vi "102_Lipgap_Full_Algo_old.vi"(0 "Image":T3(plugin-control), 1 "Calibrated Image":T3, 2 "Reference ROI":T1 {"Contours"."Type" items=["No Selection", "Point", "Line", "Rectangle", "Oval", "Polygon", "Freehand Region", "Annulus", "Unused2", "Unused3", "Broken Line", "Freehand Line", "Rotated Rectangle"]}, 3 "Line Options ROI Ref":T7={"Number of Lines"=1, "Type"=enum."First Edge Rake", "Min. Score"=10.0, "Max. Score"=1000.0, "Orientation"=0.0, "Angle Range"=45.0, "Angle Tolerance"=1.0, "Step Size"=3, "Min. SNR (db)"=0.0, "Min. Points (%)"=25.0, "Hough Iterations"=5} {"Min. Points (%)" min=0.0 max=100.0; "Min. SNR (db)" min=0.0; "Max. Score" min=0.0 max=1024.0; "Min. Score" min=0.0 max=1024.0 step=1.0}, 4 "Edge Options ROI Ref":T4={"Edge Polarity"=0, "Kernel Size"=3, "Width"=3, "Minimum Edge Strength"=50.0, "Interpolation Type"=enum."Zero Order", "Data Processing Method"=enum."Average"} {"Edge Polarity" items=["All Edges", "Rising Edges", "Falling Edges"]; "Minimum Edge Strength" format="%.2f"; "Width" step=2; "Kernel Size" step=2}, 5 "Search Direction ROI Ref":u32=3, 6 "Measurement ROI 1":T1 {"Contours"."Type" items=["No Selection", "Point", "Line", "Rectangle", "Oval", "Polygon", "Freehand Region", "Annulus", "Unused2", "Unused3", "Broken Line", "Freehand Line", "Rotated Rectangle"]}, 7 "error in (no error)":errorcluster, 8 "Blob Center":cluster{"Center X":dbl, "Center Y":dbl}, 9 "Search Direction ROI 1":u16(ring)=2 items=["Left To Right", "Right To Left", "Top To Bottom", "Bottom To Top"], 10 "Edge Options ROI 1":T4={"Edge Polarity"=0, "Kernel Size"=3, "Width"=3, "Minimum Edge Strength"=50.0, "Interpolation Type"=enum."Zero Order", "Data Processing Method"=enum."Average"} {"Edge Polarity" items=["All Edges", "Rising Edges", "Falling Edges"]; "Minimum Edge Strength" format="%.2f"; "Width" step=2; "Kernel Size" step=2}, 11 "Measurement ROI 2":T1 {"Contours"."Type" items=["No Selection", "Point", "Line", "Rectangle", "Oval", "Polygon", "Freehand Region", "Annulus", "Unused2", "Unused3", "Broken Line", "Freehand Line", "Rotated Rectangle"]}, 13 "Edge Options ROI 2":T4={"Edge Polarity"=0, "Kernel Size"=3, "Width"=3, "Minimum Edge Strength"=10.0, "Interpolation Type"=enum."Bilinear Fixed", "Data Processing Method"=enum."Average"} {"Edge Polarity" items=["All Edges", "Rising Edges", "Falling Edges"]; "Minimum Edge Strength" format="%.2f"; "Width" step=2; "Kernel Size" step=2}, 14 "Process ROI 2":T6(ring)=enum."Get All Edges", 15 "Step Size ROI 2":u32=5) -> (20 "Real World Lip Gap 102":sgl, 21 "102 Lip Gap cluster out":T2 {"102 Lip Gap ROI out"."Contours"."Type" items=["No Selection", "Point", "Line", "Rectangle", "Oval", "Polygon", "Freehand Region", "Annulus", "Unused2", "Unused3", "Broken Line", "Freehand Line", "Rotated Rectangle"]}, 27 "error IO":errorcluster)   [LabVIEW 2015]
uses:
  <vilib>/vision/Measure.llb/Straight Edge Options.ctl
  <vilib>/vision/Measure.llb/Straight Edge Process.ctl
  <vilib>/vision/Measure.llb/Edge Options.ctl
  <vilib>/vision/Measure.llb/Edge Polarity.ctl
  <vilib>/vision/Image Controls.llb/IMAQ Image.ctl
  SubVI/Clamp.llb/Find Min Max Position.vi
  <vilib>/vision/NI_Vision_Development_Module.lvlib
  FrameworkOverrides/Algorithm.lvclass
panel:
  out "Array":i32[](array[numeric])
  out "min value":sgl
  out "max value":sgl
  out "x/y":sgl
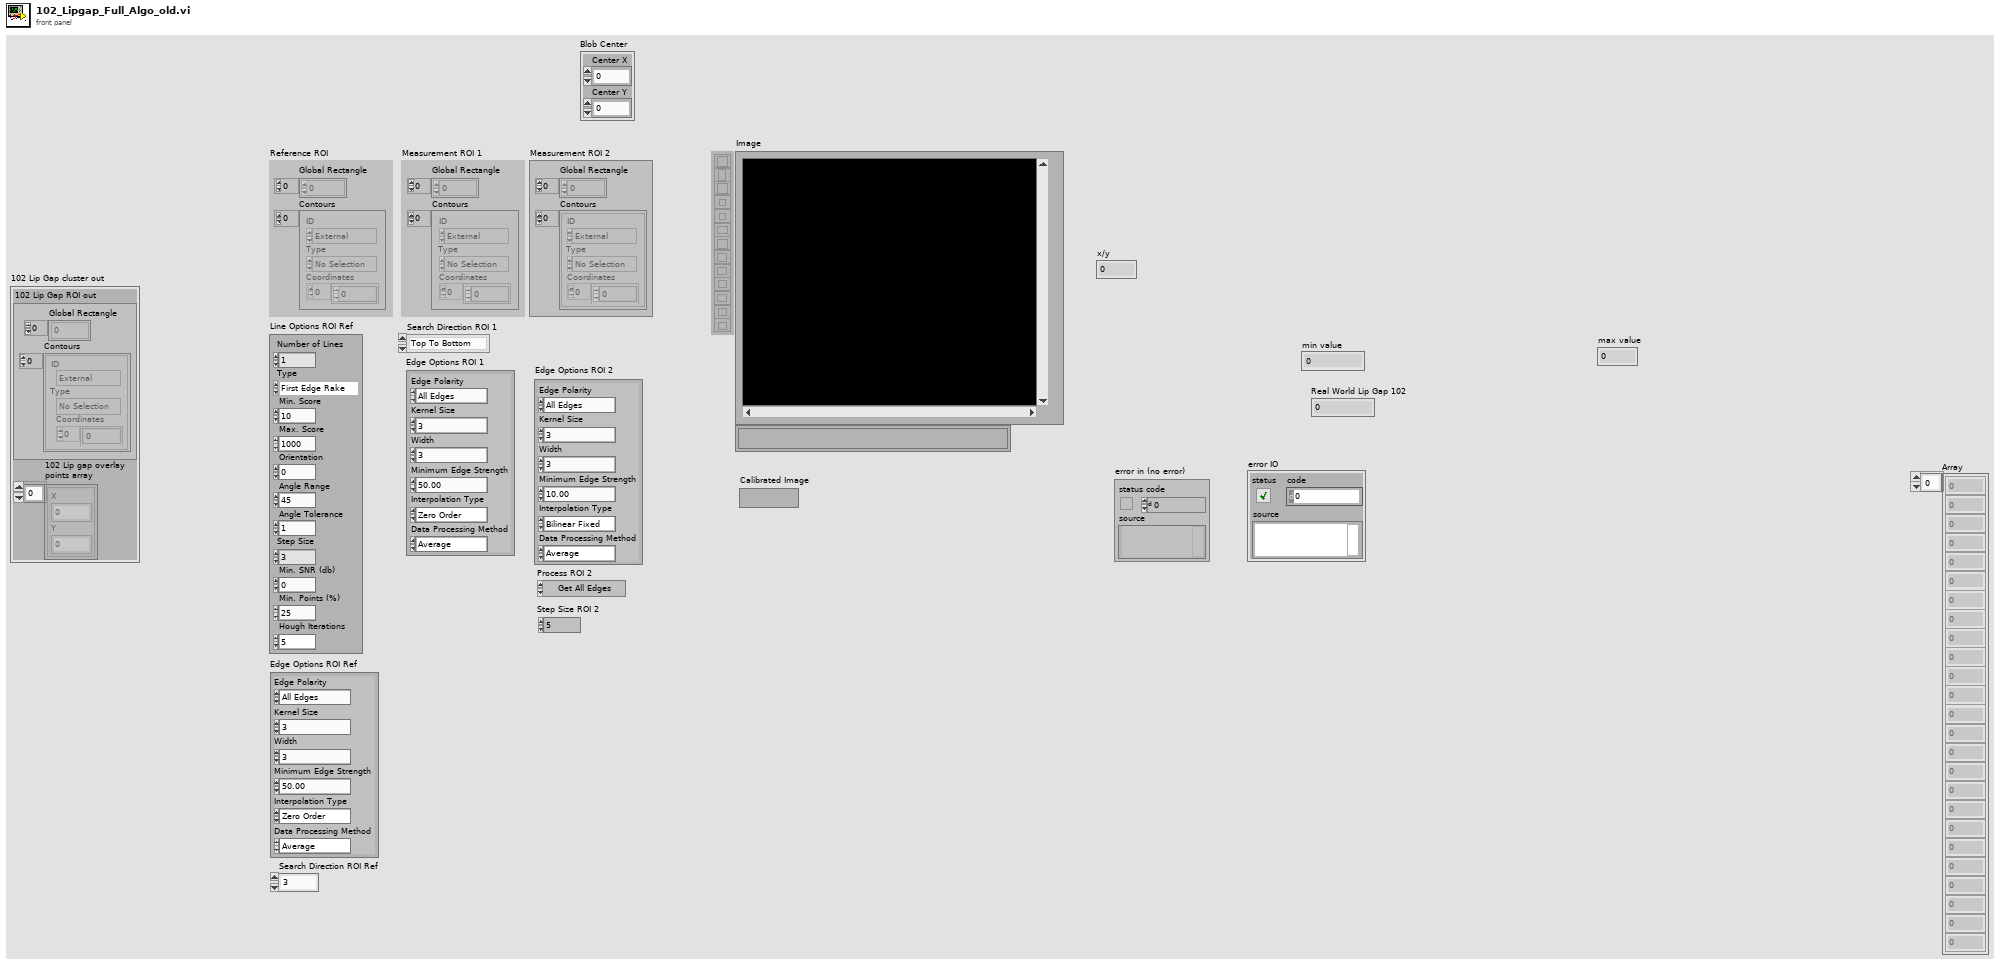
[diagram p1: front panel]
types:
  T1 = typedef "ROI Descriptor" = cluster{"Global Rectangle":i32[], "Contours":cluster{"ID":enum32{"External", "Internal"}, "Type":u32, "Coordinates":i32[]}[]}
  T2 = cluster{"102 Lip Gap ROI out":T1, "102 Lip gap overlay\npoints array":cluster{"X":sgl, "Y":sgl}[]}
  T3 = typedef "IMAQ Image.ctl" = refnum<image>
  T4 = typedef "Edge Options.ctl" = cluster{"Edge Polarity":T5, "Kernel Size":u32, "Width":u32, "Minimum Edge Strength":sgl, "Interpolation Type":enum32{"Zero Order", "Bilinear", "Quadratic", "Cubic", "Bilinear Fixed"}, "Data Processing Method":enum32{"Average", "Median"}}
  T5 = typedef "Edge Polarity.ctl" = u32
  T6 = enum16{"Get First Edge", "Get First + Last Edge", "Get All Edges", "Get Best Edge"}
  T7 = typedef "Straight Edge Options.ctl" = cluster{"Number of Lines":i32, "Type":T8, "Min. Score":dbl, "Max. Score":dbl, "Orientation":dbl, "Angle Range":dbl, "Angle Tolerance":dbl, "Step Size":u32, "Min. SNR (db)":dbl, "Min. Points (%)":dbl, "Hough Iterations":i32}
  T8 = typedef "Straight Edge Process.ctl" = enum32{"First Edge Rake", "Best Edge Rake", "Hough Edge Rake", "First Edge Projection", "Best Edge Projection"}
  T9 = typedef "IMAQ Rectangle" = cluster{"Left":i32, "Top":i32, "Right":i32, "Bottom":i32, "Rotation":dbl}
  T10 = cluster{"Left":dbl, "Top":dbl, "Right":dbl, "Bottom":dbl, "Angle":dbl}
  T11 = cluster{"Search Direction":u32, "Edge Options":T4, "Show Search Area":bool, "Show Search Lines":bool, "Show Edges Found":bool, "Show Result":bool, "Search Area Color":u32, "Search Lines Color":u32, "Edge Locations Color":u32, "Result Color":u32, "Overlay Group Name":string}
  T12 = cluster{"Point1 (Pixels)":cluster{"X":sgl, "Y":sgl}, "Point2 (Pixels)":cluster{"X":sgl, "Y":sgl}, "Point1 (Real-World)":cluster{"X":sgl, "Y":sgl}, "Point2 (Real-World)":cluster{"X":sgl, "Y":sgl}, "Angle (Pixel)":dbl, "Angle (Real-World)":dbl, "Score":dbl, "Straightness":dbl, "Average SNR (db)":dbl, "Calibration Valid":bool}[]
  T13 = cluster{"Point1 (Pixels)":cluster{"X":sgl, "Y":sgl}, "Point2 (Pixels)":cluster{"X":sgl, "Y":sgl}, "Point1 (Real-World)":cluster{"X":sgl, "Y":sgl}, "Point2 (Real-World)":cluster{"X":sgl, "Y":sgl}, "Angle (Pixel)":dbl, "Angle (Real-World)":dbl, "Score":dbl, "Straightness":dbl, "Average SNR (db)":dbl, "Calibration Valid":bool}
  T14 = typedef "IMAQ Line" = cluster{"Start X":i32, "Start Y":i32, "End X":i32, "End Y":i32}
  T15 = typedef "Search Line.ctl" = cluster{"Start Point":cluster{"X":sgl, "Y":sgl}, "End Point":cluster{"X":sgl, "Y":sgl}, "Edge Info":T16[], "Edge Map":dbl[], "Calibration Valid":bool}
  T16 = typedef "Edge New.ctl" = cluster{"Location (Pixel)":cluster{"X":sgl, "Y":sgl}, "Location (Real-World)":cluster{"X":sgl, "Y":sgl}, "Distance (Pixel)":dbl, "Distance (Real-World)":dbl, "Strength":dbl, "Noise":dbl, "Rising?":bool}
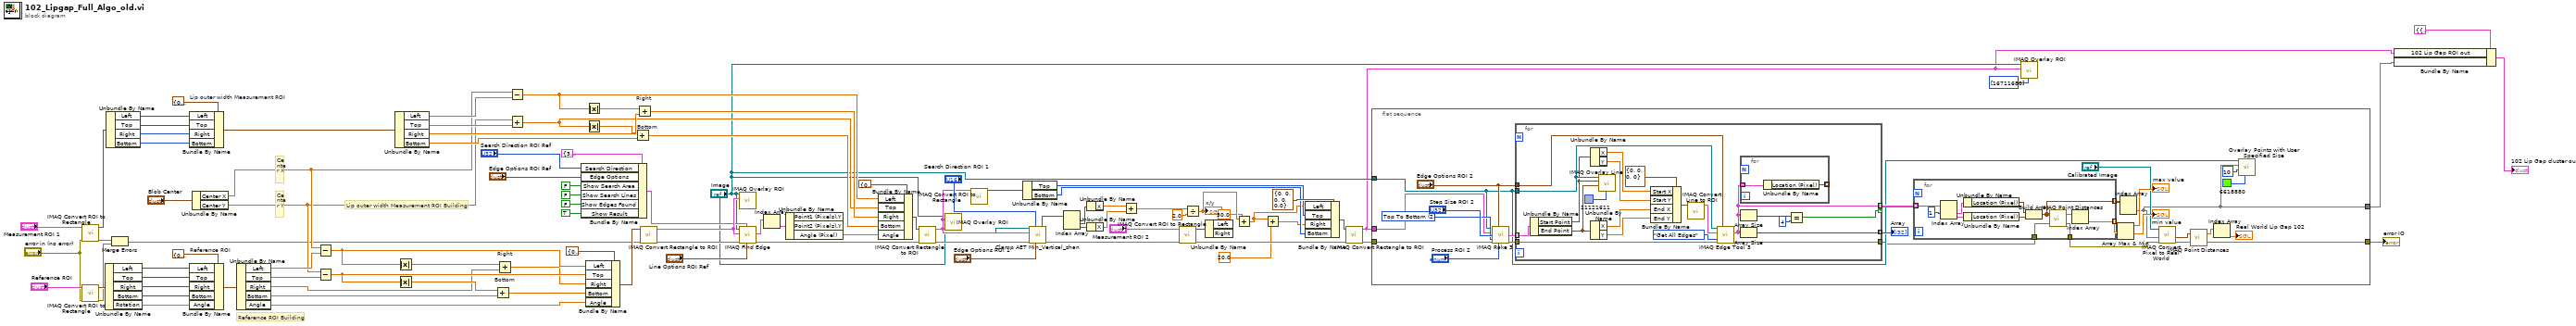
[diagram p0: block diagram]
diagram:
  # "Lip outer width Measurement ROI Building"
  # "Reference ROI Building"
  # "Center Y"
  # "Center X"
  n1 = call "IMAQ Convert ROI to Rectangle"("error in (no error)"="error in (no error)", "ROI Descriptor"="Measurement ROI 1") -> ("error out"=w45:errorcluster, "Rectangle"=w56:T9)  [unwired: 7 in]
  n2 = call "IMAQ Convert ROI to Rectangle"("error in (no error)"="error in (no error)", "ROI Descriptor"="Reference ROI") -> ("error out"=w44:errorcluster, "Rectangle"=w51:T9)  [unwired: 7 in]
  n3 = Unbundle By Name(w51) -> ("Left"=w50:i32, "Top"=w49:i32, "Right"=w48:i32, "Bottom"=w47:i32, "Rotation"=w46:dbl)
  n4 = Unbundle By Name(w56) -> ("Left"=w55:i32, "Top"=w54:i32, "Right"=w53:i32, "Bottom"=w52:i32)
  n5 = Merge Errors(w45, w44) -> (w43:errorcluster)
  n6 = Bundle By Name "Lip outer width Measurement ROI"(cluster=T10 {"Left"=0.0, "Top"=0.0, "Right"=0.0, "Bottom"=0.0, "Angle"=0.0} ("input cluster"), "Left"=w55, "Top"=w54, "Right"=w53, "Bottom"=w52) -> (w64:T10)
  n7 = Bundle By Name "Reference ROI"(cluster=T10 {"Left"=0.0, "Top"=0.0, "Right"=0.0, "Bottom"=0.0, "Angle"=0.0} ("input cluster"), "Left"=w50, "Top"=w49, "Right"=w48, "Bottom"=w47, "Angle"=w46) -> (w63:T10)
  n8 = Unbundle By Name("Blob Center") -> ("Center X"=w58:dbl, "Center Y"=w57:dbl)
  n9 = Unbundle By Name(w63) -> ("Left"=w90:dbl, "Top"=w89:dbl, "Right"=w88:dbl, "Bottom"=w87:dbl, "Angle"=w86:dbl)
  n10 = Subtract(x=w58, y=w90) -> (x-y=w94:dbl)
  n11 = Subtract(x=w57, y=w89) -> (x-y=w93:dbl)
  n12 = Unbundle By Name(w64) -> ("Left"=w73:dbl, "Top"=w72:dbl, "Right"=w71:dbl, "Bottom"=w70:dbl)
  n13 = Absolute Value(x=w94) -> (abs(x)=w97:dbl)
  n14 = Absolute Value(x=w93) -> (abs(x)=w96:dbl)
  n15 = Add "Bottom"(x=w96, y=w87) -> (x+y=w91:dbl)
  n16 = Add "Right"(x=w97, y=w88) -> (x+y=w92:dbl)
  n17 = Subtract(x=w58, y=w73) -> (x-y=w76:dbl)
  n18 = Add(x=w57, y=w72) -> (x+y=w68:dbl)
  n19 = Bundle By Name(cluster=T11 {"Search Direction"=3, "Edge Options"={"Edge Polarity"=0, "Kernel Size"=3, "Width"=3, "Minimum Edge Strength"=50.0, "Interpolation Type"=enum."Zero Order", "Data Processing Method"=enum."Average"}, "Show Search Area"=FALSE, "Show Search Lines"=FALSE, "Show Edges Found"=FALSE, "Show Result"=TRUE, "Search Area Color"=65280, "Search Lines Color"=255, "Edge Locations Color"=16776960, "Result Color"=16711680, "Overlay Group Name"=""} ("Options"), "Search Direction"="Search Direction ROI Ref", "Edge Options"="Edge Options ROI Ref", "Show Search Area"=FALSE, "Show Search Lines"=FALSE, "Show Edges Found"=FALSE, "Show Result"=TRUE) -> (w38:T11)
  n20 = Absolute Value(x=w76) -> (abs(x)=w78:dbl)
  n21 = Absolute Value(x=w68) -> (abs(x)=w69:dbl)
  n22 = Bundle By Name(cluster=T10 {"Left"=0.0, "Top"=0.0, "Right"=0.0, "Bottom"=0.0, "Angle"=0.0} ("input cluster"), "Left"=w94, "Top"=w93, "Right"=w92, "Bottom"=w91, "Angle"=w86) -> (w81:T10)
  n23 = Add "Bottom"(x=w69, y=w70) -> (x+y=w74:dbl)
  n24 = Add "Right"(x=w78, y=w71) -> (x+y=w75:dbl)
  n25 = call "IMAQ Convert Rectangle to ROI"("error in (no error)"=w43, "Rectangle"=w81) -> ("error out"=w85:errorcluster, "ROI Descriptor"=w79:T1)  [unwired: 7 in]
  n26 = call "IMAQ Overlay ROI"("ROI Descriptor"=w79, "Image"="Image") -> ()  [unwired: 8 in, 2 out]
  n27 = call "IMAQ Find Edge"("Line Fit Options"="Line Options ROI Ref", "Options"=w38, "error in (no error)"=w85, "ROI Descriptor"=w79, "Image"="Image") -> ("error out"=w42:errorcluster, "Straight Edges"=w83:T12)  [unwired: 3 in, 2 out]
  n28 = Index Array(array=w83) -> (element=w82:T13)  [unwired: 1 in]
  n29 = Unbundle By Name(w82) -> ("Angle (Pixel)"=w66:dbl)  [unwired: 2 out]
  n30 = Bundle By Name(cluster=T10 {"Left"=0.0, "Top"=0.0, "Right"=0.0, "Bottom"=0.0, "Angle"=0.0} ("input cluster"), "Left"=w76, "Top"=w68, "Right"=w75, "Bottom"=w74, "Angle"=w66) -> (w67:T10)
  n31 = call "IMAQ Convert Rectangle to ROI"("error in (no error)"=w42, "Rectangle"=w67) -> ("error out"=w62:errorcluster, "ROI Descriptor"=w23:T1)  [unwired: 7 in]
  n32 = call "IMAQ Overlay ROI"("ROI Descriptor"=w23, "Image"="Image") -> ()  [unwired: 8 in, 2 out]
  n33 = call "IMAQ Convert ROI to Rectangle"("ROI Descriptor"=w23) -> ("Rectangle"=w22:T9)  [unwired: 8 in, 1 out]
  n34 = Unbundle By Name(w22) -> ("Top"=w20:i32, "Bottom"=w19:i32)
  n35 = call "Clamp AET Min_Vertical_shan.vi"("Image"="Image", "Scanning axis"="Search Direction ROI 1", "ROI Descriptor"=w23, "error in (no error)"=w62, "Edge Options"="Edge Options ROI 1") -> ("Edge Coordinates"=w31:cluster{"X":sgl, "Y":sgl}[], "error out"=w10:errorcluster)  [unwired: 3 in, 6 out]
  n36 = Index Array(array=w31) -> (element #1=w30:cluster{"X":sgl, "Y":sgl}, element #2=w29:cluster{"X":sgl, "Y":sgl})  [unwired: 2 in]
  n37 = Unbundle By Name(w30) -> ("X"=w28:sgl)
  n38 = Unbundle By Name(w29) -> ("X"=w27:sgl)
  n39 = Add(x=w28, y=w27) -> (x+y=w26:sgl)
  n40 = call "IMAQ Convert ROI to Rectangle"("error in (no error)"=w10, "ROI Descriptor"="Measurement ROI 2") -> ("error out"=w9:errorcluster, "Rectangle"=w12:T9)  [unwired: 7 in]
  n41 = Divide(x=w26, y=sgl 2.0) -> (x/y=w24:sgl)
  "x/y" <- w24
  n42 = Unbundle By Name(w12) -> ()  [unwired: 2 out]
  n43 = Add(x=w24, y=sgl 30.0) -> (x+y=w18:sgl)
  n44 = Add(x=w18, y=sgl 20.0) -> (x+y=w17:sgl)
  n45 = Bundle By Name(cluster=T9 {"Left"=0, "Top"=0, "Right"=0, "Bottom"=0, "Rotation"=0.0} ("Rectangle"), "Left"=w18, "Top"=w20, "Right"=w17, "Bottom"=w19) -> (w16:T9)
  n46 = call "IMAQ Convert Rectangle to ROI"("error in (no error)"=w9, "Rectangle"=w16) -> ("error out"=w13:errorcluster, "ROI Descriptor"=w2:T1)  [unwired: 7 in]
  n47 = flat-sequence {
    tunnel: "Image" -> [w101]
    tunnel: w2 -> [w107]
    tunnel: w13 -> [w106]
    tunnel: [w104] -> w7
    tunnel: [w98] -> w1
    frame #0 {
      w122 = u16 2 items=["Left To Right", "Right To Left", "Top To Bottom", "Bottom To Top"] ("Scan Direction ROI 2")
      n48 = call "IMAQ Rake 3"("Image"=w101, "Edge Options"="Edge Options ROI 2", "ROI Descriptor"=w107, "Step Size"="Step Size ROI 2", "Scan Direction"=w122, "error in (no error)"=w106, "Process"="Process ROI 2") -> ("Search Lines"=w120:T15[], "error out"=w118:errorcluster)  [unwired: 5 in, 2 out]
      n49 = for {
        tunnel: w120 -> [w155] mode=indexing
        tunnel: w101 -> [w144]
        tunnel: "Edge Options ROI 2" -> [w145]
        tunnel: w118 -> [w143]
        tunnel: [w142] -> w100
        tunnel: [w139] -> w117 mode=indexing
        tunnel: [w138] -> w116 mode=indexing if=w135
        n50 = Unbundle By Name(w155) -> ("Start Point"=w141:cluster{"X":sgl, "Y":sgl}, "End Point"=w140:cluster{"X":sgl, "Y":sgl})
        n51 = Unbundle By Name(w141) -> ("X"=w152:sgl, "Y"=w151:sgl)
        n52 = Unbundle By Name(w140) -> ("X"=w150:sgl, "Y"=w149:sgl)
        n53 = call "IMAQ Overlay Line"("Color"=u32 11121611, "End Point"=w140, "Start Point"=w141, "Image"=w144) -> ()  [unwired: 6 in, 2 out]
        n54 = Bundle By Name(cluster=T14 {"Start X"=0, "Start Y"=0, "End X"=0, "End Y"=0} ("Line"), "Start X"=w152, "Start Y"=w151, "End X"=w150, "End Y"=w149) -> (w148:T14)
        n55 = call "IMAQ Convert Line to ROI"("Line"=w148) -> ("ROI Descriptor"=w147:T1)  [unwired: 8 in, 1 out]
        n56 = call "IMAQ Edge Tool 3"("Image"=w144, "Edge Options"=w145, "ROI Descriptor"=w147, "Process"=T6."Get All Edges", "error in (no error)"=w143) -> ("Edge Information"=w138:T16[], "error out"=w142:errorcluster)  [unwired: 6 in, 3 out]
        n57 = for {
          tunnel: w138 -> [w157] mode=indexing
          tunnel: [w156] -> _ mode=indexing
          n58 = Unbundle By Name(w157) -> ("Location (Pixel)"=w156:cluster{"X":sgl, "Y":sgl})
        }
        n59 = Array Size(array=w138) -> (size(s)=w137:i32)
        n60 = Array Size(array=w138) -> (size(s)=w139:i32)
        n61 = Equal?(x=w137, y=4) -> (x = y?=w135:bool)
      }
      "Array" <- w117
      n62 = for {
        tunnel: w116 -> [w134] mode=indexing
        tunnel: [w127] -> w115 mode=indexing
        tunnel: [w126] -> w112 mode=indexing
        tunnel: w100 -> [w125]
        tunnel: [w124] -> w99
        n63 = Index Array(array=w134, index #1=1 ("index")) -> (element #1=w132:T16, element #2=w131:T16)  [unwired: 1 in]
        n64 = Unbundle By Name(w132) -> ("Location (Pixel)"=w130:cluster{"X":sgl, "Y":sgl})
        n65 = Unbundle By Name(w131) -> ("Location (Pixel)"=w129:cluster{"X":sgl, "Y":sgl})
        n66 = Build Array(w130, w129) -> (w126:cluster{"X":sgl, "Y":sgl}[])
        n67 = call "IMAQ Point Distances"("Points"=w126, "error in (no error)"=w125) -> ("Distances"=w128:sgl[], "error out"=w124:errorcluster)  [unwired: 3 in]
        n68 = Index Array(array=w128) -> (element=w127:sgl)  [unwired: 1 in]
      }
      n69 = Array Max & Min(array=w115) -> (max value=→"max value":sgl, min value=→"min value":sgl)  [unwired: 2 out]
      n70 = Index Array(array=w112) -> (element=w98:cluster{"X":sgl, "Y":sgl}[])  [unwired: 2 in]
      n71 = call "IMAQ Convert Pixel to Real World"("error in (no error)"=w99, "Array of Pixel Coordinates"=w98, "Calibrated Image"="Calibrated Image") -> ("error out"=w110:errorcluster, "Array of Real World Coordinates"=w111:cluster{"X":sgl, "Y":sgl}[])  [unwired: 3 in, 4 out]
      n72 = call "IMAQ Point Distances"("Points"=w111, "error in (no error)"=w110) -> ("Distances"=w109:sgl[], "error out"=w104:errorcluster)  [unwired: 3 in]
      n73 = Index Array(array=w109) -> (element=→"Real World Lip Gap 102":sgl)  [unwired: 1 in]
      n74 = call "Overlay Points with User Specified Size.vi"("Color"=u32 6618880, "Point Diameter (5)"=u32 10, "Points"=w98, "Image In"=w101) -> ()  [unwired: 6 in, 2 out]
    }
  }
  n75 = call "IMAQ Overlay ROI"("Colors (Green)"=u32[] [16711680], "ROI Descriptor"=w2, "Image"="Image") -> ()  [unwired: 7 in, 2 out]
  n76 = Bundle By Name(cluster=T2 {"102 Lip Gap ROI out"={"Global Rectangle"=[], "Contours"=[]}, "102 Lip gap overlay\npoints array"=[]} ("102 Lip Gap cluster out"), "102 Lip Gap ROI out"=w2, "102 Lip gap overlay\npoints array"=w1) -> (→"102 Lip Gap cluster out":T2)
  "error IO" <- w7
